vi "Data Directory File Count,Size Limiter.vi"(7 "File Count Limit (2000)":u16=2000, 8 "error in":errorcluster, 9 "Data Storage Limit(104,857,600 bytes = 100MB)":i64=104857600 format="%.0p", 10 "Data Storage Pattern":string="*.dat", 11 "Data Storage Path":path) -> (0 "error out":errorcluster, 1 "Data storage used before deletions":i64 format="%.0p", 2 "Data File List":string[](array[string]), 3 "Files Removed":i64)   [LabVIEW 2011]
doc: "This VI searches for a set of data storage files at a specified path and limits the total amount of disk space they utilize. Files will be deleted from oldest to newest until the specified limit is achieved.\n\nThe data file names must be in ascending order by date (oldest-newest).\nFor example:s\nDataFile 2010-12-30 09-46-33.dat\nDataFile 2010-12-30 09-49-53.dat\nDataFile 2010-12-30 10-02-41.dat, etc.\n\n\nVersion 1.0 - 2/13/2013\n\nPhaeron, Inc.\nwww.phaeron.com\ninfo@phaeron.com"
panel:
  out "# Files":i32
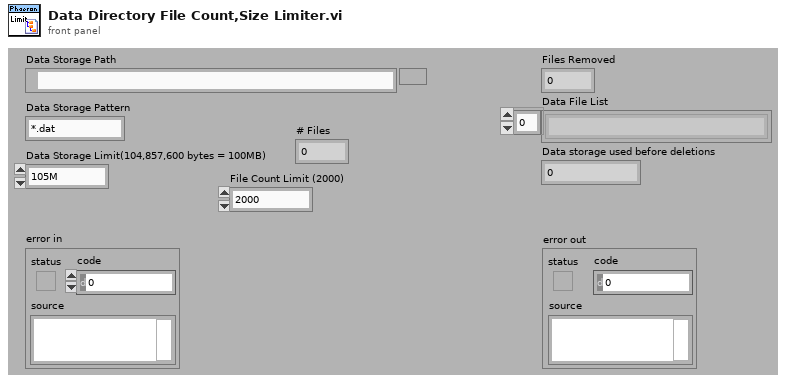
[diagram p1: front panel]
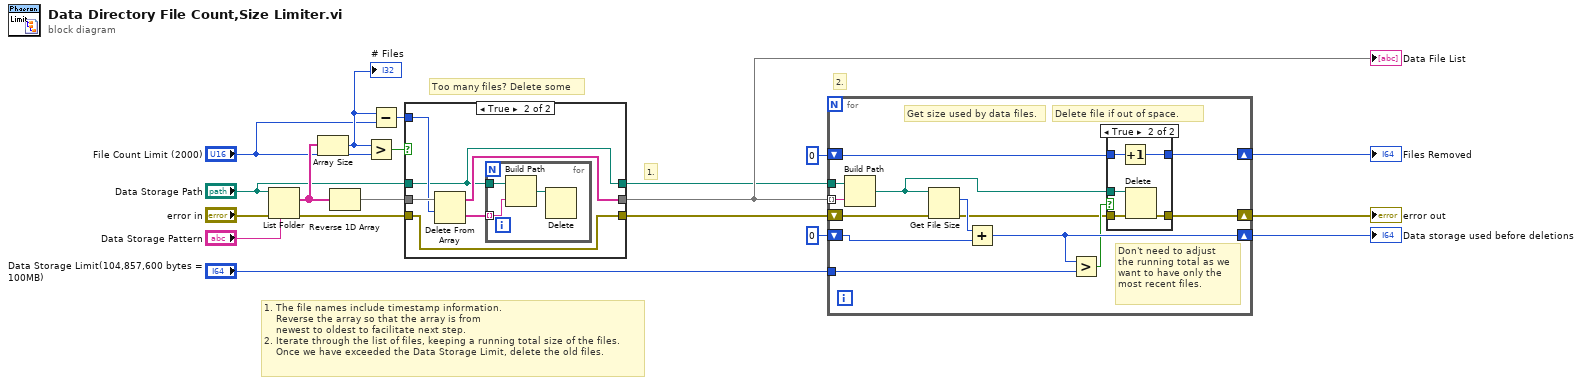
[diagram p0: block diagram]
diagram:
  # "2."
  # "Too many files? Delete some"
  # "1. The file names include timestamp information.\n    Reverse the array so that the array is from\n    newest to oldest to facilitate next step.\n2. Iterate through the list of files, keeping a running total size of the files.\n    Once we have exceeded the Data Storage Limit, delete the old files."
  # "1."
  n1 = List Folder(path="Data Storage Path", pattern="Data Storage Pattern", error in="error in") -> (filenames=w14:string[], error out=w8:errorcluster)  [unwired: 1 in, 2 out]
  n2 = Array Size(array=w14) -> (size(s)=w7:i32)
  "# Files" <- w7
  n3 = Reverse 1D Array(array=w14) -> (reversed array=w12:string[])
  n4 = Greater?(x=w7, y="File Count Limit (2000)") -> (0:w10:bool)
  n5 = Subtract(x=w7, y="File Count Limit (2000)") -> (x-y=w5:i32)
  n6 = case shown="True" w10 {
    tunnel: "Data Storage Path" -> [w22 w24]
    tunnel: w12 -> [w21 w28]
    tunnel: [w21 w26] -> w11
    tunnel: [w22 w24] -> w3
    tunnel: [w20 w23] -> w9
    tunnel: w8 -> [w20 w23]
    tunnel: w5 -> [_ w27]
    frame False {
    }
    frame True {
      n7 = Delete From Array(array=w28, length=w27) -> (deleted portion=w25:string[], array with subset deleted=w26:string[])  [unwired: 1 in]
      n8 = for {
        tunnel: w24 -> [w31]
        tunnel: w25 -> [w29] mode=indexing
        n9 = Build Path(base path=w31, name or relative path=w29) -> (appended path=w30:path)
        n10 = Delete(path (use dialog)=w30) -> ()  [unwired: 4 in, 3 out]
      }
    }
  }
  "Data File List" <- w11
  n11 = for {
    tunnel: w11 -> [w43] mode=indexing
    tunnel: w3 -> [w44]
    shift-right: [w40] -> w18
    shift-left: i64 0 -> [w41]
    tunnel: "Data Storage Limit(104,857,600 bytes = 100MB)" -> [w39]
    shift-right: [w34] -> w17
    shift-left: w9 -> [w38]
    shift-right: [w32] -> w16
    shift-left: i64 0 -> [w33]
    # "Don't need to adjust\nthe running total as we\nwant to have only the\nmost recent files."
    # "Delete file if out of space."
    # "Get size used by data files."
    n12 = Build Path(base path=w44, name or relative path=w43) -> (appended path=w36:path)
    n13 = Get File Size(file=w36, error in=w38) -> (size (in bytes)=w42:i64, 0:w35:errorcluster)  [unwired: 1 out]
    n14 = Add(x=w42, y=w41) -> (x+y=w40:i64)
    n15 = Greater?(x=w40, y=w39) -> (0:w37:bool)
    n16 = case shown="True" w37 {
      tunnel: w36 -> [_ w51]
      tunnel: w35 -> [w46 w50]
      tunnel: [w46 w49] -> w34
      tunnel: w33 -> [w45 w48]
      tunnel: [w45 w47] -> w32
      frame False {
      }
      frame True {
        n17 = Increment(x=w48) -> (x+1=w47:i64)
        n18 = Delete(path (use dialog)=w51, error in=w50) -> (error out=w49:errorcluster)  [unwired: 3 in, 2 out]
      }
    }
  }
  "Data storage used before deletions" <- w18
  "error out" <- w17
  "Files Removed" <- w16
